vi "const all vi refs.vi"() -> (3 "initial pool sizes":T1)   [LabVIEW 2013, in "thread pool.lvclass"]
uses:
  thread pool.lvclass
  task/task.lvclass
  task/strict executor reference.ctl
  vi references.ctl
  DAQ executor.vi
  Instrument IO executor.vi
  other 2 executor.vi
  standard executor.vi
  UI executor.vi
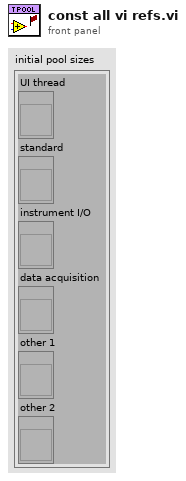
[diagram p1: front panel]
types:
  T1 = typedef "thread pool.lvclass/vi references.ctl" = cluster{"UI thread":T2, "standard":T2, "instrument I/O":T2, "data acquisition":T2, "other 1":T2, "other 2":T2}
  T2 = typedef "thread pool.lvclass/strict executor reference.ctl" = refnum<vi>
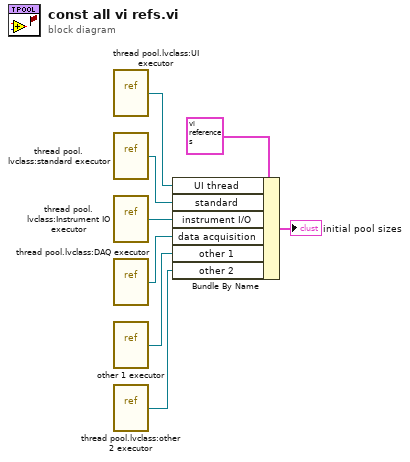
[diagram p0: block diagram]
diagram:
  n1 = vi-ref "thread pool.lvclass:UI executor.vi"() -> (w2:refnum<vi>)
  n2 = vi-ref "thread pool.lvclass:standard executor.vi"() -> (w3:refnum<vi>)
  n3 = vi-ref "thread pool.lvclass:Instrument IO executor.vi"() -> (w4:refnum<vi>)
  n4 = vi-ref "thread pool.lvclass:DAQ executor.vi"() -> (w5:refnum<vi>)
  n5 = vi-ref "other 1 executor.vi"() -> (w6:refnum<vi>)
  n6 = vi-ref "thread pool.lvclass:other 2 executor.vi"() -> (w1:refnum<vi>)
  n7 = Bundle By Name(cluster=T1 {"UI thread"=refnum, "standard"=refnum, "instrument I/O"=refnum, "data acquisition"=refnum, "other 1"=refnum, "other 2"=refnum} ("initial pool sizes"), "UI thread"=w2, "standard"=w3, "instrument I/O"=w4, "data acquisition"=w5, "other 1"=w6, "other 2"=w1) -> (→"initial pool sizes":T1)
